vi "HatchStateControl.vi"(9 "Elevator State":string, 10 "Vacuum Pump Power":dbl) -> ()   [LabVIEW 2018]
uses:
  RobotStates.vi
  Inputs_DriverStation.vi
panel:
  in  "HATCH Eject Time (ms)":u32=1000
  in  "Vacuum Pump Off Time (ms)":u32=2000
  in  "Suction Cup Pulse (ms)":u32=100
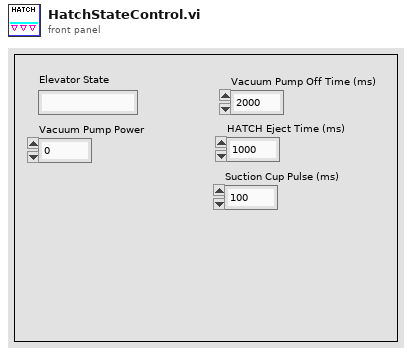
[diagram p1: front panel]
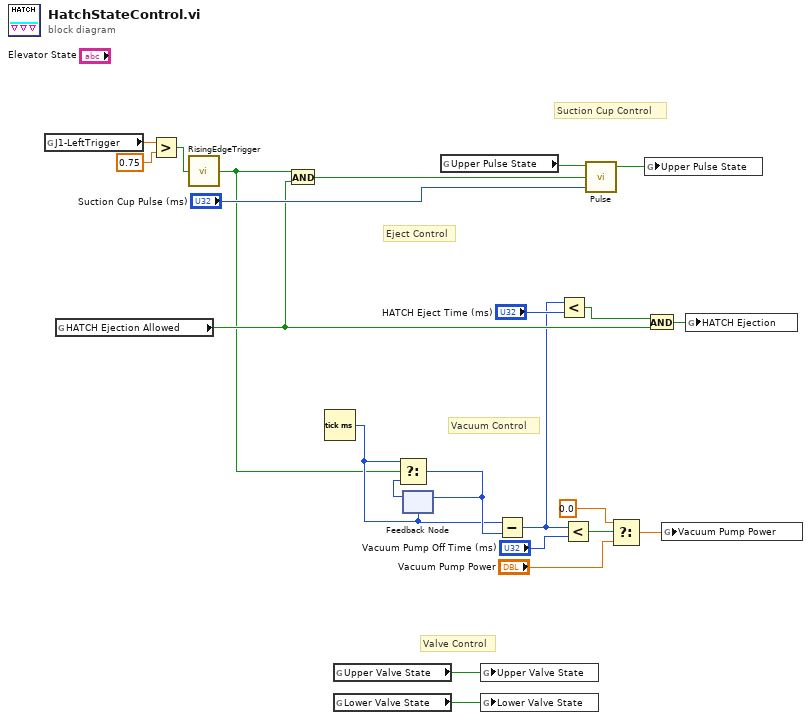
[diagram p0: block diagram]
diagram:
  # "Valve Control"
  # "Eject Control"
  # "Vacuum Control"
  # "Suction Cup Control"
  n1 = global read "Inputs_DriverStation.vi" "J1-LeftTrigger"() -> (w10:dbl)
  n2 = global read "RobotStates.vi" "HATCH Ejection Allowed"() -> (w6:bool)
  n3 = Greater?(x=w10, y=0.75) -> (0:w11:bool)
  n4 = call "RisingEdgeTrigger.vi"("Raw Signal"=w11) -> ("Trigger"=w1:bool)
  n5 = And(x=w1, y=w6) -> (x .and. y?=w7:bool)
  n6 = Tick Count (ms)() -> (millisecond timer value=w18:u32)
  n7 = global read "RobotStates.vi" "Upper Valve State"() -> (w13:bool)
  n8 = global read "RobotStates.vi" "Lower Valve State"() -> (w12:bool)
  n9 = feedback #1(w18) -> (w20:u32)
  n10 = Select(t=w18, s=w1, f=w20) -> (s? t:f=w19:u32)
  n11 = feedback-in #1(w19) -> ()
  n12 = global read "RobotStates.vi" "Upper Pulse State"() -> (w22:bool)
  n13 = global write "RobotStates.vi" "Upper Valve State"(w13) -> ()
  n14 = global write "RobotStates.vi" "Lower Valve State"(w12) -> ()
  n15 = Subtract(x=w18, y=w19) -> (x-y=w3:u32)
  n16 = Less?(x=w3, y="HATCH Eject Time (ms)") -> (x < y?=w2:bool)
  n17 = Less?(x=w3, y="Vacuum Pump Off Time (ms)") -> (x < y?=w5:bool)
  n18 = call "Pulse.vi"("Pulse Duration (ms)"="Suction Cup Pulse (ms)", "Trigger"=w7, "State In"=w22) -> ("State Out"=w21:bool)  [unwired: 2 in]
  n19 = Select(t=0.0, s=w5, f="Vacuum Pump Power") -> (s? t:f=w14:dbl)
  n20 = global write "RobotStates.vi" "Upper Pulse State"(w21) -> ()
  n21 = And(x=w2, y=w6) -> (x .and. y?=w8:bool)
  n22 = global write "RobotStates.vi" "Vacuum Pump Power"(w14) -> ()
  n23 = global write "RobotStates.vi" "HATCH Ejection"(w8) -> ()
